vi "Set NVMEM Bytes.vi"(0 "SLSC Remote in":refnum<class "SLSC Remote.lvclass">, 5 "NVMEM area":refnum<k21>="$DefaultNVMEMAreas", 7 "data address":u32 format="%.0x", 9 "data":u8[](array[numeric]) format="%.0x", 11 "error in (no error)":errorcluster) -> (4 "SLSC Remote out":refnum<class "SLSC Remote.lvclass">, 6 "NVMEM area out":refnum<k21>, 8 "next data address":u32 format="%.0x", 15 "error out":errorcluster)   [LabVIEW 2016, in "SLSC Interfaces.lvlib" / "SLSC Remote.lvclass"]
uses:
  SLSC Remote.lvclass
  C:/Users/tblair/Documents/SLSC-Interface/Source/SLSC Interface Class/SLSC Interface.lvclass
  <vilib>/rajsite/i3-json/JSON Generation/Create Value Files/Create Value - Object.vi
  <vilib>/rajsite/i3-json/JSON Generation/Add Object Parameter Files/Add Object Parameter - String.vi
  <vilib>/rajsite/i3-json/JSON Generation/Add Object Parameter Files/Add Object Parameter - Numeric.vi
  <vilib>/rajsite/i3-json/JSON Generation/Add Object Parameter Files/Add Object Parameter - 1D Array Double.vi
  <vilib>/NI/NI JSONRPC Server Framework/Classes/Server/Format Client Request (Auto-Increment).vi
  <vilib>/httpClient/POSTBuffer.vi
  <vilib>/rajsite/i3-json/JSON Parsing/Get Object Parameter Files/Get Object Parameter - Numeric.vi
  <vilib>/NI/NI JSONRPC Server Framework/Classes/Server/JSONRPC Server.lvclass
  <vilib>/rajsite/i3-json/i3-json.lvlib
  <vilib>/httpClient/LabVIEWHTTPClient.lvlib
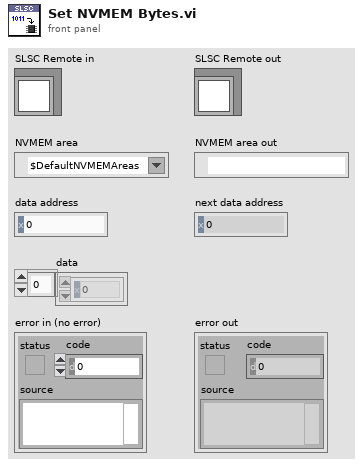
[diagram p1: front panel]
types:
  T1 = typedef "LabVIEWHTTPClient.lvlib/ClientHandle.ctl" = refnum<k1>
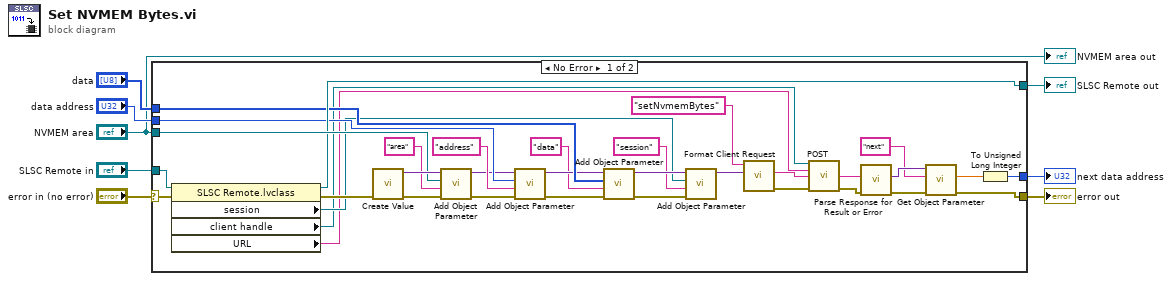
[diagram p0: block diagram]
diagram:
  n1 = case shown="No Error" "error in (no error)" {
    selector: "error in (no error)" -> [w36 w44]
    tunnel: "NVMEM area" -> [w41 _]
    tunnel: [w39 w43] -> w2
    tunnel: "data address" -> [w37 _]
    tunnel: "data" -> [w32 _]
    tunnel: [w11 w44] -> w1
    tunnel: "SLSC Remote in" -> [w15 w43]
    tunnel: [w9 _] -> w8
    frame No Error {
      n2 = property class="SLSC Remote.lvclass"(reference=w15, error in=w36) -> (reference out=w39:refnum<class "SLSC Remote.lvclass">, error out=w35:errorcluster, "session"=w24:refnum<k21>, "client handle"=w22:T1, "URL"=w21:string)
      n3 = call-poly <vilib>:"Create Value.vi"("error in (no error)"=w35) -> ("error out"=w34:errorcluster, "JSON Tree"=w42:variant)  [unwired: 9 in]
      n4 = call-poly <vilib>:"Add Object Parameter.vi"("error in (no error)"=w34, "Name"="area", "String"=w41, "JSON Tree in (JSON Object)"=w42) -> ("error out"=w33:errorcluster, "JSON Tree out (JSON Object)"=w29:variant)  [unwired: 6 in]
      n5 = call-poly <vilib>:"Add Object Parameter.vi"("error in (no error)"=w33, "Name"="address", "Numeric"=w37, "JSON Tree in (JSON Object)"=w29) -> ("error out"=w27:errorcluster, "JSON Tree out (JSON Object)"=w28:variant)  [unwired: 6 in]
      n6 = call-poly <vilib>:"Add Object Parameter.vi"("error in (no error)"=w27, "Name"="data" ("String"), "1D Double"=w32, "JSON Tree in (JSON Object)"=w28) -> ("error out"=w25:errorcluster, "JSON Tree out (JSON Object)"=w26:variant)  [unwired: 6 in]
      n7 = call-poly <vilib>:"Add Object Parameter.vi"("error in (no error)"=w25, "Name"="session", "String"=w24, "JSON Tree in (JSON Object)"=w26) -> ("JSON Tree out (JSON Object)"=w16:variant)  [unwired: 6 in, 1 out]
      n8 = call-poly <vilib>:"Format Client Request.vi"("params"=w16, "method"="setNvmemBytes") -> ("error out"=w20:errorcluster, "Request String"=w30:string)  [unwired: 8 in]
      n9 = call-poly <vilib>:"POST.vi"("client handle"=w22, "url"=w21, "buffer"=w30, "error in (no error)"=w20) -> ("body"=w18:string, "error out"=w17:errorcluster)  [unwired: 8 in, 2 out]
      n10 = call <vilib>:"Parse Response for Result or Error.vi"("error in"=w17, "Response String In"=w18) -> ("error out"=w12:errorcluster, "Result or Error Data"=w14:variant)  [unwired: 7 in, 1 out]
      n11 = call-poly <vilib>:"Get Object Parameter.vi"("error in (no error)"=w12, "Parameter Name"="next", "JSON Tree In (JSON Object)"=w14) -> ("error out"=w11:errorcluster, "Double Value"=w10:dbl)  [unwired: 5 in, 2 out]
      n12 = To Unsigned Long Integer(number=w10) -> (unsigned 32bit integer=w9:u32)
    }
    frame Error {
    }
  }
  "error out" <- w1
  "SLSC Remote out" <- w2
  "next data address" <- w8
  "NVMEM area out" <- "NVMEM area"
